vi "FGV Leak Daten.vi"(0 "Gesamtvolumen":T4 {"LeakValve" items=["inactive", "active"]}, 5 "Dichtheitstest aktiv":bool, 7 "Dichtheitstest Zustand":T3, 9 "Leak Protokoll":T1={"Bearbeiter:"="", "Pfad:"=path "D:/IAG_Data/Log", "Textname:"="", "Analysator"=""} caption="T90 Konfig Daten", 11 "error in (no error)":errorcluster caption="Fehler (Eingang, kein Fehler)", 13 "Aktion":T5) -> (4 "Gesamtvolumen":T4 {"LeakValve" items=["inactive", "active"]}, 6 "Dichtheitstest aktiv":bool, 8 "Dichtheitstest Zustand":T3, 10 "Leak Protokoll":T1={"Bearbeiter:"="", "Pfad:"=path "D:/IAG_Data/Log", "Textname:"="", "Analysator"=""} caption="T90 Konfig Daten", 15 "error out":errorcluster caption="Fehler (Ausgang)")   [LabVIEW 2020, in "EPA 1065.lvlib" / "Dichtheitstest 1065-345.lvlib"]
uses:
  Dichtheitstest 1065-345.lvlib
  Aktion Leak Daten.ctl
  Gesamtvolumen.ctl
  Aktion Leak check durchfuehren.ctl
  Leak Protokoll Einstellungen.ctl
  Seiten/System Einstellungen V2/Analysatoren.ctl
  Seiten/System Einstellungen V2/System Einstellungen V2.lvlib
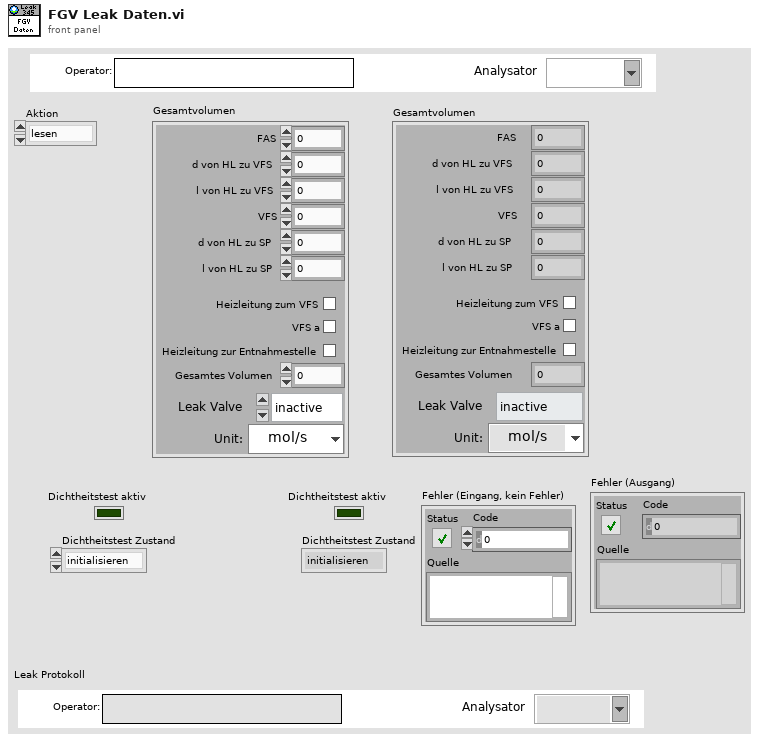
[diagram p1: front panel]
types:
  T1 = typedef "EPA 1065.lvlib/Dichtheitstest 1065-345.lvlib/Leak Protokoll Einstellungen.ctl" = cluster{"Bearbeiter:":string, "Pfad:":path, "Textname:":string, "Analysator":T2}
  T2 = typedef "System Einstellungen V2.lvlib/Analysatoren.ctl" = string
  T3 = typedef "EPA 1065.lvlib/Dichtheitstest 1065-345.lvlib/Aktion Leak check durchfuehren.ctl" = enum16{"initialisieren", "Unterdruck erzeugen", "Ventile schließen", "Warten", "Auswertung", "fertig", "PDF erstellen", "abbrechen"}
  T4 = typedef "EPA 1065.lvlib/Dichtheitstest 1065-345.lvlib/Gesamtvolumen.ctl" = cluster{"FAS":sgl, "d von HL zu VFS":sgl, "l von HL zu VFS":sgl, "VFS":sgl, "d von HL zu SP":sgl, "l von HL zu SP":sgl, "Heizleitung zum VFS":bool, "VFS a":bool, "Heizleitung zur Entnahmestelle":bool, "Gesamtes Volumen":sgl, "LeakValve":u16, "Einheit":enum16{"mol/s", "mbar"}}
  T5 = typedef "EPA 1065.lvlib/Dichtheitstest 1065-345.lvlib/Aktion Leak Daten.ctl" = enum16{"lesen", "laden", "speichern", "Volumen", "berechnen", "Leak check aktiv", "Leak Zustand", "Pfad", "Pfad speichern"}
  T6 = enum16{"laden", "speichern", "Pfad laden", "Pfad speichern"}
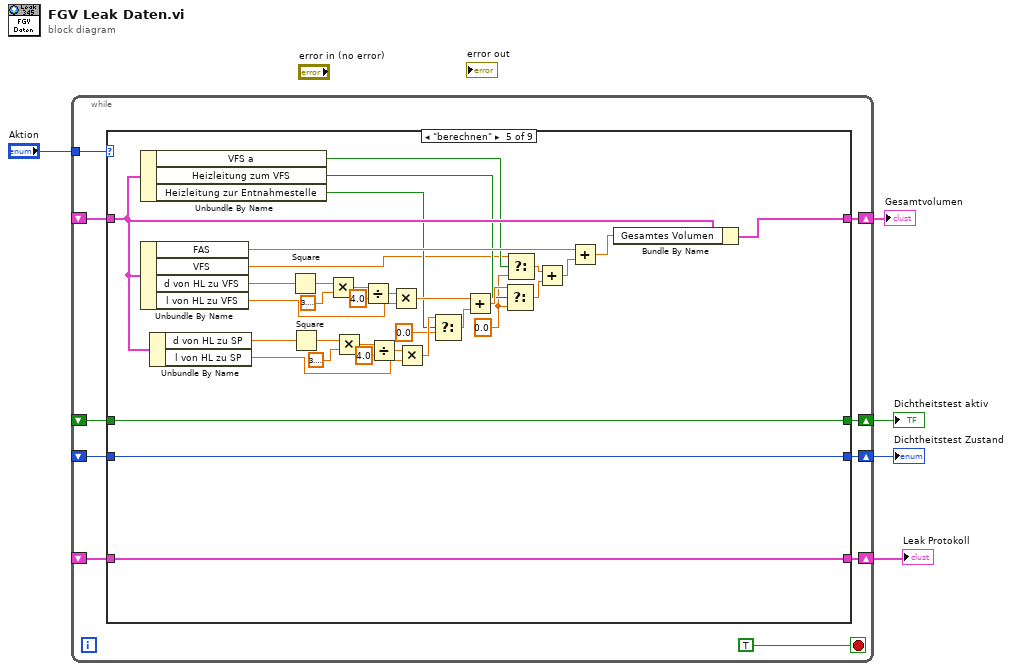
[diagram p0: block diagram]
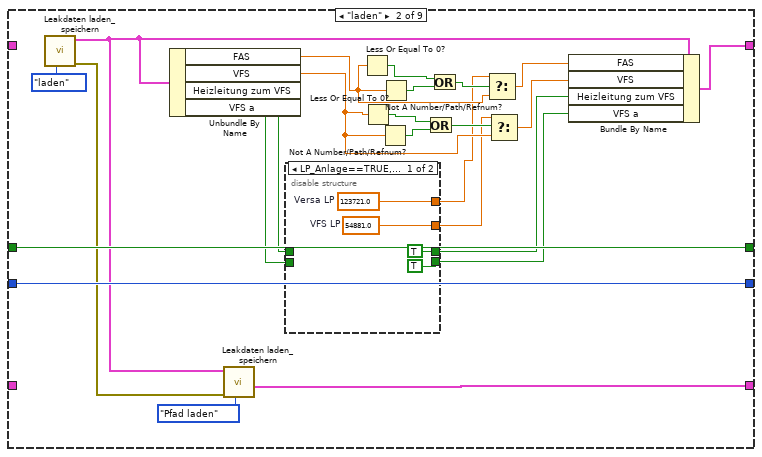
[diagram p3: hidden frame]
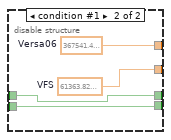
[diagram p4: hidden frame]
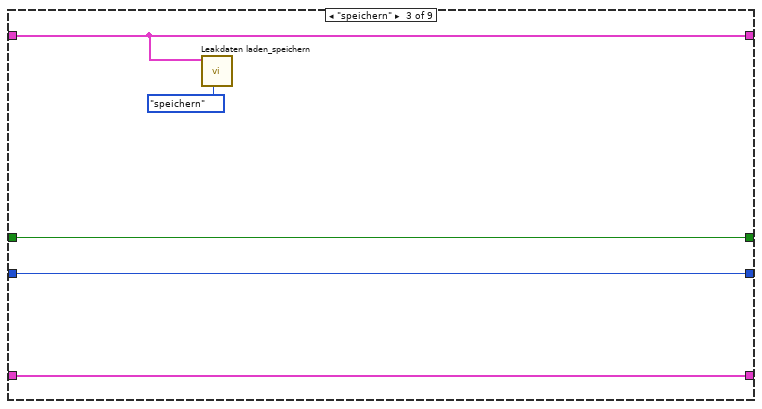
[diagram p5: hidden frame]
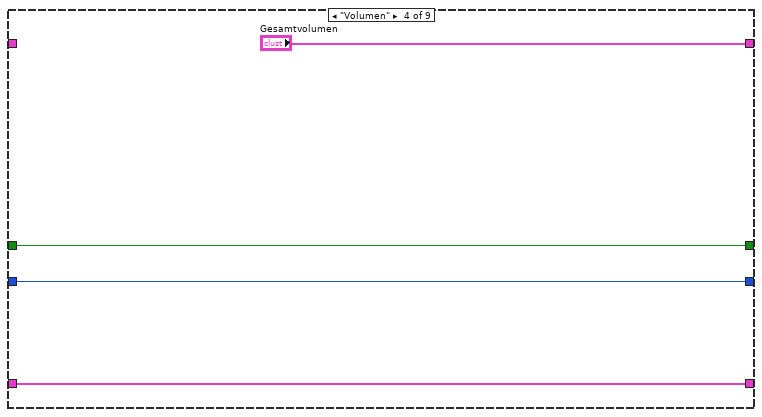
[diagram p6: hidden frame]
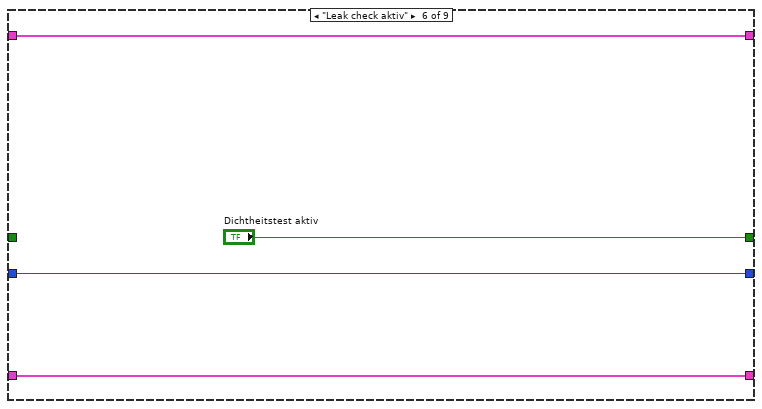
[diagram p7: hidden frame]
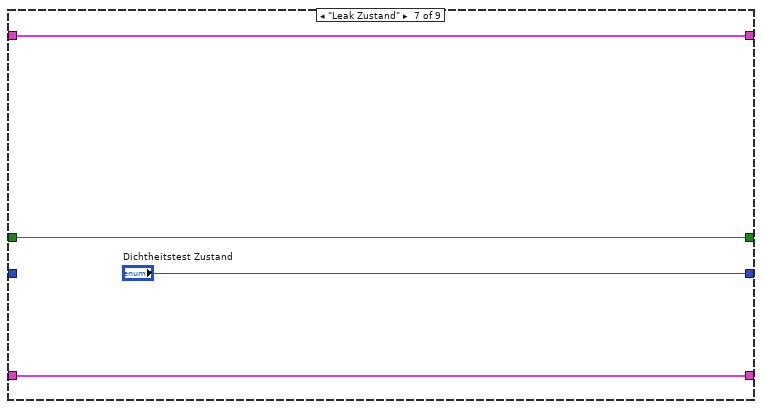
[diagram p8: hidden frame]
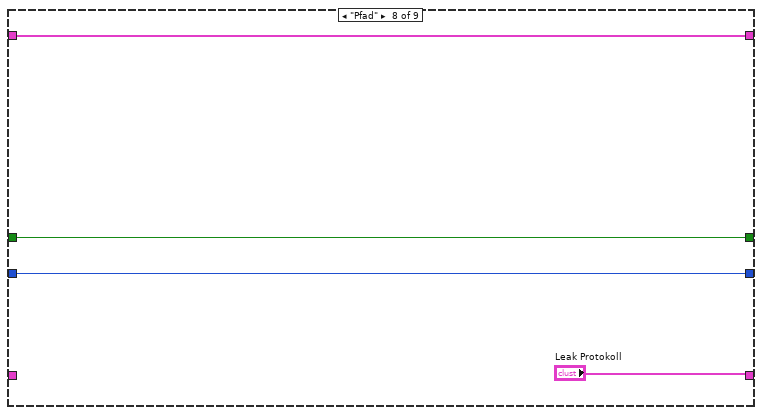
[diagram p9: hidden frame]
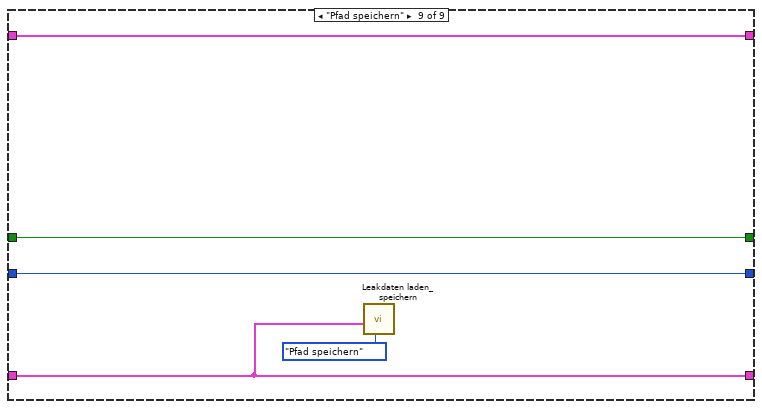
[diagram p10: hidden frame]
diagram:
  n1 = while {
    tunnel: "Aktion" -> [w14]
    shift-right: [w13] -> w4
    shift-left: _ -> [w12]
    shift-right: [w11] -> w3
    shift-left: _ -> [w10]
    shift-right: [w9] -> w2
    shift-left: _ -> [w8]
    shift-right: [w7] -> w1
    shift-left: _ -> [w6]
    stop <- TRUE stop-if-true
    n2 = case shown="\"berechnen\"" w14 {
      tunnel: [w19 w26 w56 "Gesamtvolumen" w77 w96 w100 w106 w111] -> w13
      tunnel: w12 -> [w19 _ w56 _ w73 w96 w100 w106 w111]
      tunnel: [w18 w43 w55 w59 w75 "Dichtheitstest aktiv" w101 w105 w110] -> w11
      tunnel: w10 -> [w18 w43 w55 w59 w75 _ w101 w105 w110]
      tunnel: [w17 w42 w54 w58 w74 w97 "Dichtheitstest Zustand" w104 w109] -> w9
      tunnel: w8 -> [w17 w42 w54 w58 w74 w97 _ w104 w109]
      tunnel: [w16 w39 w52 w57 w61 w95 w99 "Leak Protokoll" w107] -> w7
      tunnel: w6 -> [w16 _ w52 w57 w61 w95 w99 _ w107]
      frame "lesen", Default {
      }
      frame "laden" {
        n3 = call "Leakdaten laden_speichern.vi"("Aktion"=T6."laden") -> ("error out"=w38:errorcluster, "Gesamtvolumen"=w29:T4)  [unwired: 8 in, 1 out]
        n4 = Unbundle By Name(w29) -> ("FAS"=w31:sgl, "VFS"=w30:sgl, "Heizleitung zum VFS"=w23:bool, "VFS a"=w22:bool)
        n5 = call "Leakdaten laden_speichern.vi"("Aktion"=T6."Pfad laden", "error in (no error)"=w38, "Gesamtvolumen"=w29) -> ("Leak Protokoll"=w39:T1)  [unwired: 6 in, 2 out]
        n6 = disable-structure shown="LP_Anlage==TRUE, Standard" {
          disable-tunnel: [w47 w51] -> w25
          disable-tunnel: [w46 w50] -> w24
          disable-tunnel: w23 -> [_ w49]
          disable-tunnel: w22 -> [_ w48]
          disable-tunnel: [TRUE ("Heizleitung zum VFS") w49] -> w21
          disable-tunnel: [TRUE ("VFS a") w48] -> w20
          frame condition #0 (active) {
            w46 = sgl 54881.0  # VFS LP
            w47 = sgl 123721.0  # Versa LP
          }
          frame condition #1 {
            w50 = sgl 61363.83  # VFS
            w51 = sgl 367541.4  # Versa06
          }
        }
        n7 = Less Or Equal To 0?(x=w31) -> (x <= 0?=w36:bool)
        n8 = Less Or Equal To 0?(x=w30) -> (x <= 0?=w34:bool)
        n9 = Not A Number/Path/Refnum?(number/path/refnum=w30) -> (NaN/Path/Refnum?=w35:bool)
        n10 = Not A Number/Path/Refnum?(number/path/refnum=w31) -> (NaN/Path/Refnum?=w37:bool)
        n11 = Or(x=w34, y=w35) -> (x .or. y?=w33:bool)
        n12 = Or(x=w36, y=w37) -> (x .or. y?=w32:bool)
        n13 = Select(t=w25, s=w32, f=w31) -> (s? t:f=w28:sgl)
        n14 = Select(t=w24, s=w33, f=w30) -> (s? t:f=w27:sgl)
        n15 = Bundle By Name(cluster=w29, "FAS"=w28, "VFS"=w27, "Heizleitung zum VFS"=w21, "VFS a"=w20) -> (w26:T4)
      }
      frame "speichern" {
        n16 = call "Leakdaten laden_speichern.vi"("Aktion"=T6."speichern", "Gesamtvolumen"=w56) -> ()  [unwired: 7 in, 3 out]
      }
      frame "Volumen" {
      }
      frame "berechnen" {
        w64 = sgl 0.0 ("f")
        n17 = Unbundle By Name(w73) -> ("VFS a"=w63:bool, "Heizleitung zum VFS"=w67:bool, "Heizleitung zur Entnahmestelle"=w71:bool)
        n18 = Unbundle By Name(w73) -> ("FAS"=w79:sgl, "VFS"=w62:sgl, "d von HL zu VFS"=w93:sgl, "l von HL zu VFS"=w89:sgl)
        n19 = Unbundle By Name(w73) -> ("d von HL zu SP"=w84:sgl, "l von HL zu SP"=w88:sgl)
        n20 = Square(x=w93) -> (x^2=w94:sgl)
        n21 = Square(x=w84) -> (x^2=w82:sgl)
        n22 = Multiply(x=w94, y=sgl 3.1415927) -> (x*y=w92:sgl)
        n23 = Multiply(x=w82, y=sgl 3.1415927) -> (x*y=w85:sgl)
        n24 = Divide(x=w92, y=sgl 4.0) -> (x/y=w90:sgl)
        n25 = Divide(x=w85, y=sgl 4.0) -> (x/y=w87:sgl)
        n26 = Multiply(x=w90, y=w89) -> (x*y=w81:sgl)
        n27 = Multiply(x=w87, y=w88) -> (x*y=w72:sgl)
        n28 = Select(t=w72, s=w71, f=sgl 0.0) -> (s? t:f=w69:sgl)
        n29 = Add(x=w81, y=w69) -> (x+y=w68:sgl)
        n30 = Select(t=w68, s=w67, f=w64) -> (s? t:f=w66:sgl)
        n31 = Select(t=w62, s=w63, f=w64) -> (s? t:f=w65:sgl)
        n32 = Add(x=w65, y=w66) -> (x+y=w80:sgl)
        n33 = Add(x=w79, y=w80) -> (x+y=w76:sgl)
        n34 = Bundle By Name(cluster=w73, "Gesamtes Volumen"=w76) -> (w77:T4)
      }
      frame "Leak check aktiv" {
      }
      frame "Leak Zustand" {
      }
      frame "Pfad" {
      }
      frame "Pfad speichern" {
        n35 = call "Leakdaten laden_speichern.vi"("Aktion"=T6."Pfad speichern", "Leak Protokoll"=w107) -> ()  [unwired: 7 in, 3 out]
      }
    }
  }
  "Gesamtvolumen" <- w4
  "Dichtheitstest aktiv" <- w3
  "Dichtheitstest Zustand" <- w2
  "Leak Protokoll" <- w1
